vi "testingoutfileopener.vi"() -> ()   [LabVIEW 2020]
doc: "Use this template to build a producer/consumer design pattern. Use this template when you need to execute a process, such as data analysis, when a data source, such as a triggered acquisition, produces data at an uneven rate and you need to execute the process when the data becomes available.\n------------------------------------\nAuther: Koji Ohashi\nCopyright (c) 2020 Japan LabVIEW Users Group, Volunteer members.\nThis VI is released under the MIT License.\nhttp://opensource.org/licenses/mit-license.php\n------------------------------------"
uses:
  For fsr type def.ctl
  <vilib>/Analysis/baseanly.llb/Mean (DBL).vi
  <vilib>/Instr/_visa.llb/VISA Configure Serial Port (Instr).vi
  <vilib>/Analysis/NI_AALBase.lvlib
panel:
  in  "Folder name: Participant":string caption="Participant Name (FirstLast)"
  in  "Create/Replace file":bool
  out "Vout F4":dbl(slide) scale=0.0..5.0
  out "Collecting":bool
  in  "Timer [ms]":u32=5000
  out "On Time [ms]":u32
  out "millisecond timer":u32
  in  "Weight":T1(ring)
  out "Vout F1":dbl(slide) scale=0.0..5.0
  in  "Refresh":bool
  in  "Test Type":string
  in  "Path":path=path "C:/Users/rsKite/Documents/FSR DATA"
  in  "Trial":string caption="Participant Name (FirstLast)"
  out "File Name":string
  out "Vout F3":dbl(slide) scale=0.0..5.0
  out "Vout F2":dbl(slide) scale=0.0..5.0
  out "Status":string
  in  "Collect":bool
  in  "VISA resource name":refnum<visa-resource-name>="COM1"
  in  "stop":bool
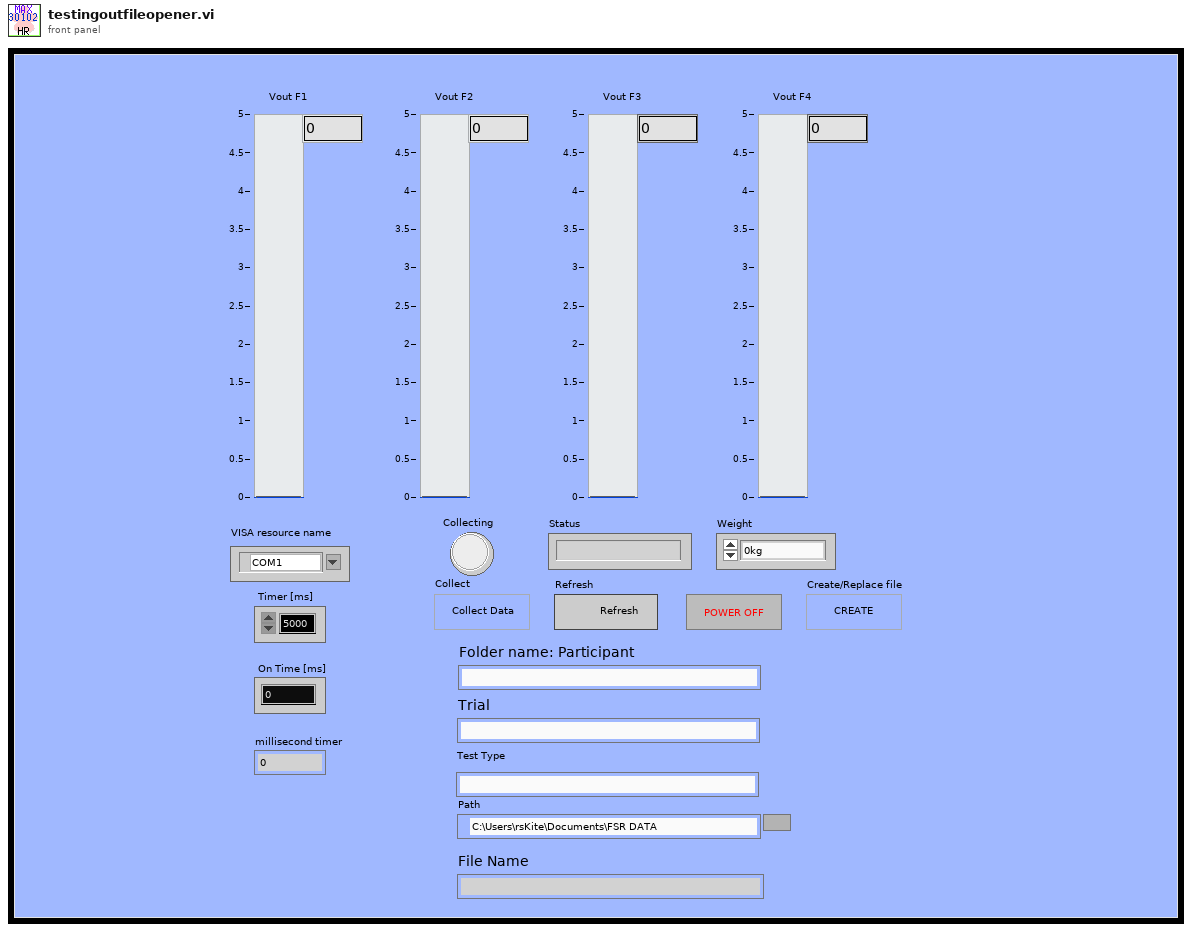
[diagram p1: front panel]
types:
  T1 = enum16{"0kg", "0.1kg", "0.2kg", "0.3kg", "0.4kg", "0.5kg", "0.6kg", "0.7kg", "0.8kg", "0.9kg", "1kg", "1.1kg", "1.2kg", "1.3kg", "1.4kg", "1.5kg", "1.6kg", "1.7kg", "1.8kg", "1.9kg", "2.0kg"}
  T2 = typedef "For fsr type def.ctl" = enum16{"Create/Replace File", "Waiting Room", "Collect Data", "Write Data", "Close File", "Reinit"}
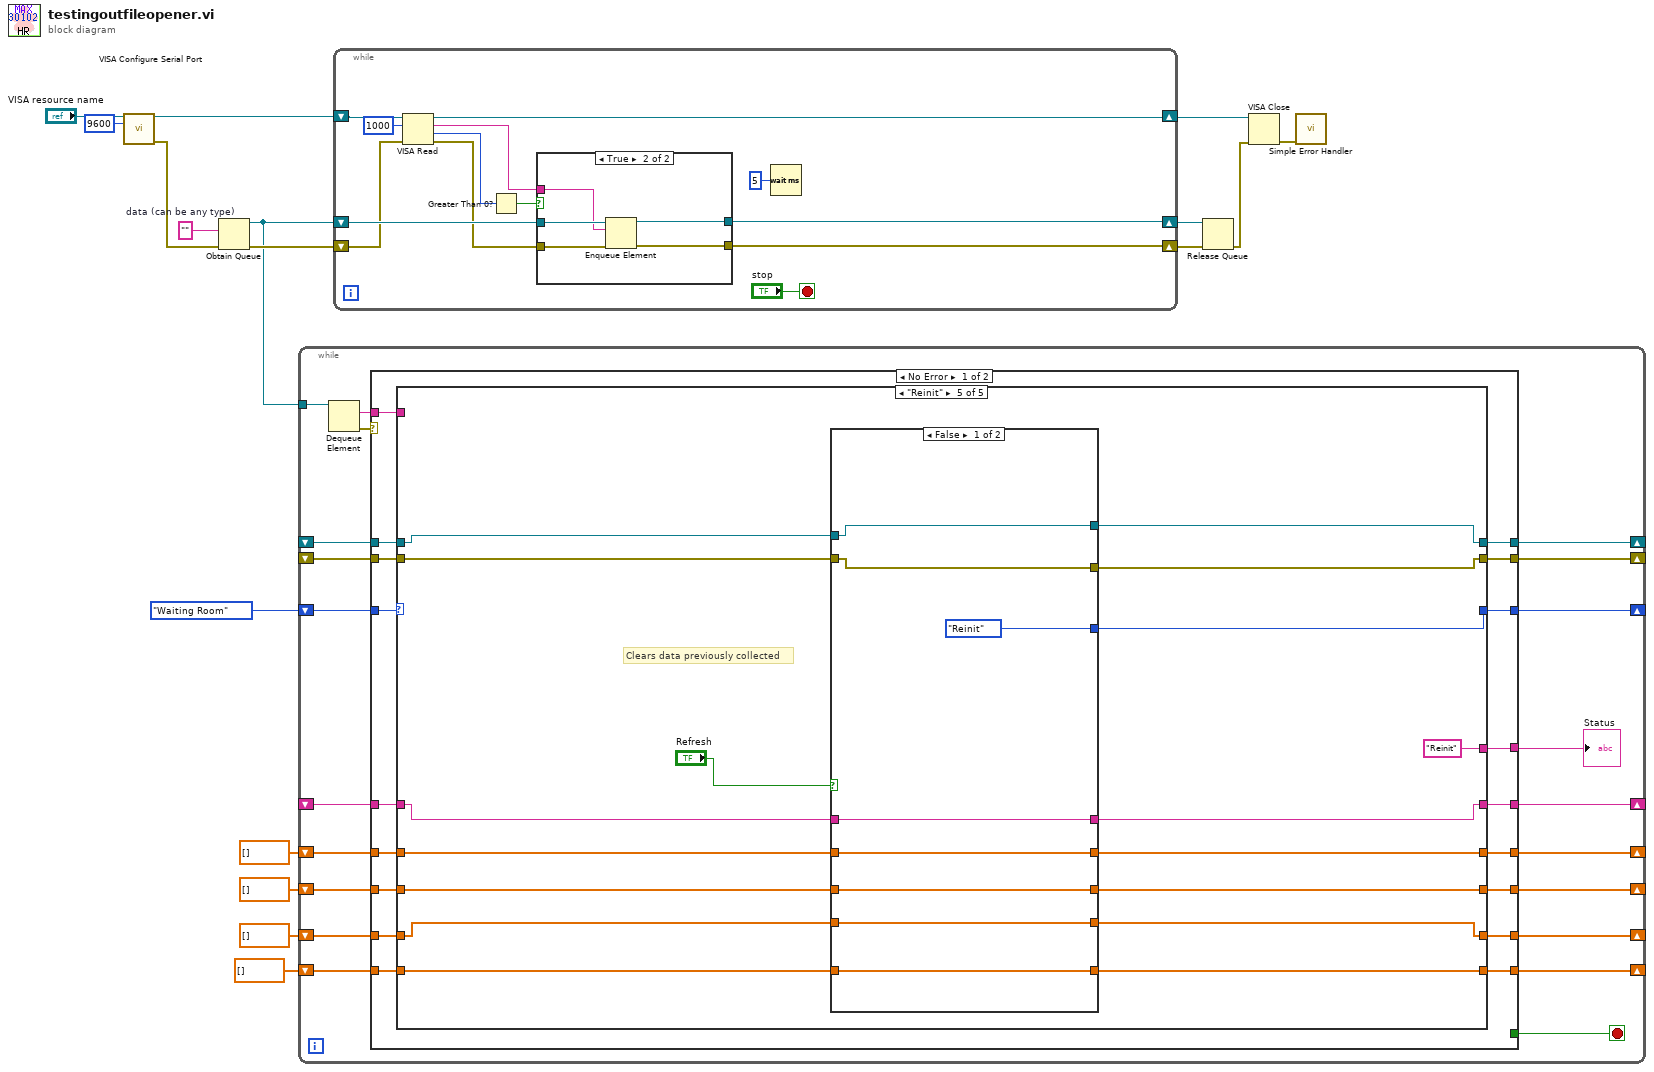
[diagram p0: block diagram]
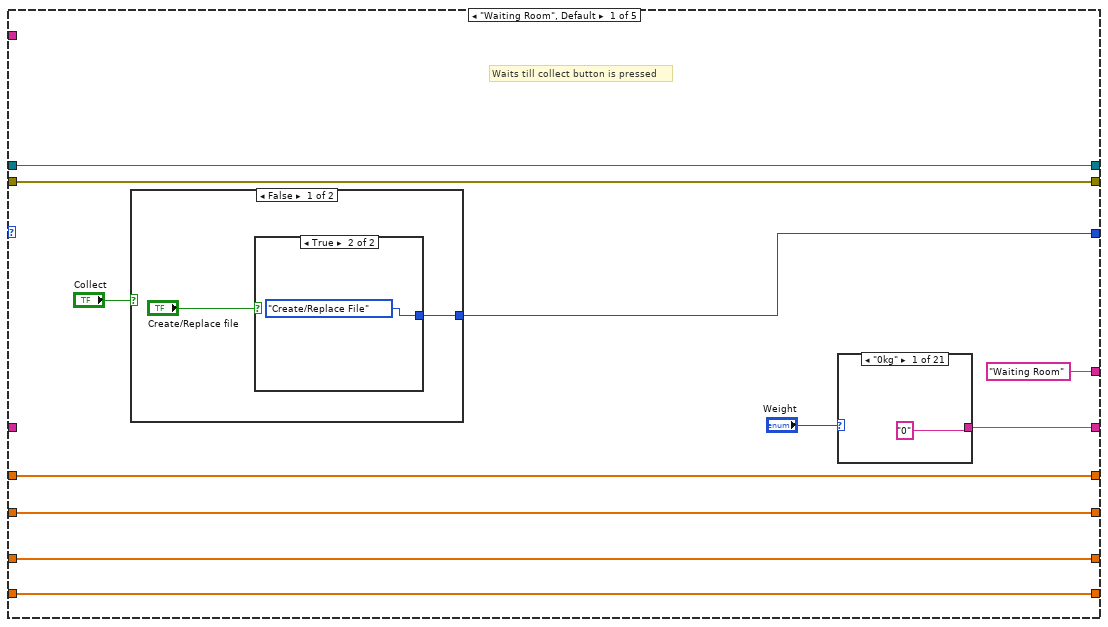
[diagram p2: hidden frame]
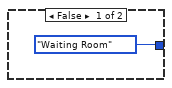
[diagram p3: hidden frame]
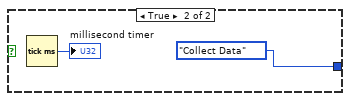
[diagram p4: hidden frame]
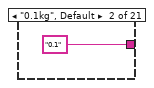
[diagram p5: hidden frame]
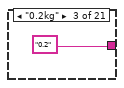
[diagram p6: hidden frame]
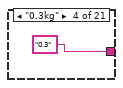
[diagram p7: hidden frame]
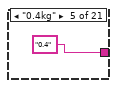
[diagram p8: hidden frame]
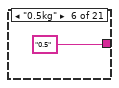
[diagram p9: hidden frame]
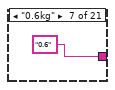
[diagram p10: hidden frame]
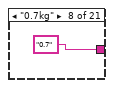
[diagram p11: hidden frame]
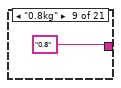
[diagram p12: hidden frame]
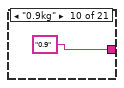
[diagram p13: hidden frame]
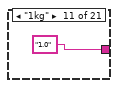
[diagram p14: hidden frame]
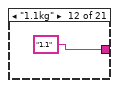
[diagram p15: hidden frame]
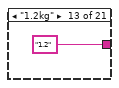
[diagram p16: hidden frame]
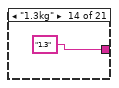
[diagram p17: hidden frame]
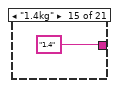
[diagram p18: hidden frame]
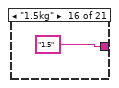
[diagram p19: hidden frame]
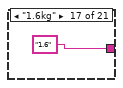
[diagram p20: hidden frame]
diagram:
  w14 = ""  # data (can be any type)
  n1 = call-poly "VISA Configure Serial Port"("VISA resource name"="VISA resource name", "baud rate (9600)"=u32 9600) -> ("VISA resource name out"=w12:refnum<visa-resource-name>, "error out"=w9:errorcluster)  [unwired: 8 in, 4 out]
  n2 = Obtain Queue(element data type=w14, error in (no error)=w9) -> (queue out=w1:refnum<queue>, error out=w17:errorcluster)  [unwired: 3 in, 1 out]
  n3 = while {
    tunnel: w1 -> [w38]
    shift-right: [w33] -> _
    shift-left: For_fsr_type_def."Waiting Room" -> [w34]
    shift-right: [w29] -> _
    shift-left: dbl[] [] -> [w30]
    shift-right: [w31] -> _
    shift-left: dbl[] [] -> [w32]
    shift-right: [w27] -> _
    shift-left: dbl[] [] -> [w28]
    shift-right: [w25] -> _
    shift-left: _ -> [w26]
    shift-right: [w23] -> _
    shift-left: dbl[] [] -> [w24]
    shift-right: [w21] -> _
    shift-left: _ -> [w19]
    shift-right: [w20] -> _
    shift-left: _ -> [w18]
    stop <- w22 stop-if-true
    n4 = Dequeue Element(queue=w38) -> (element=w36:string, error out=w37:errorcluster)  [unwired: 2 in, 2 out]
    n5 = case shown="No Error" w37 {
      tunnel: w36 -> [w54 _]
      tunnel: [w53 "Error or POWER OFF"] -> w35
      tunnel: w34 -> [w56 _]
      tunnel: [w55 For_fsr_type_def."Waiting Room"] -> w33
      tunnel: w32 -> [w52 w213]
      tunnel: [w51 w213] -> w31
      tunnel: w30 -> [w50 w214]
      tunnel: [w49 w214] -> w29
      tunnel: w28 -> [w48 w215]
      tunnel: [w47 w215] -> w27
      tunnel: w26 -> [w46 w212]
      tunnel: [w45 w212] -> w25
      tunnel: w24 -> [w44 w211]
      tunnel: [w43 w211] -> w23
      tunnel: [_ TRUE] -> w22
      tunnel: [w42 w209] -> w21
      tunnel: [w41 w208] -> w20
      tunnel: w19 -> [w40 w209]
      tunnel: w18 -> [w39 w208]
      frame No Error {
        n6 = case shown="\"Reinit\"" w56 {
          tunnel: [w59 For_fsr_type_def."Waiting Room" w112 For_fsr_type_def."Reinit" w184] -> w55
          tunnel: w54 -> [_ _ w138 _ _]
          tunnel: ["Waiting Room" "Creating" "Collect data" "Write Data" "Reinit"] -> w53
          tunnel: w52 -> [w64 w98 w134 w162 w179]
          tunnel: [w64 w98 w119 w162 w188] -> w51
          tunnel: w50 -> [w65 w99 w131 w163 w180]
          tunnel: [w65 w99 w129 w163 w187] -> w49
          tunnel: w48 -> [w66 w101 w130 w164 w181]
          tunnel: [w66 w101 w128 w164 w186] -> w47
          tunnel: [w63 w100 w126 w154 w185] -> w45
          tunnel: w46 -> [_ w100 w126 w154 w182]
          tunnel: w44 -> [w61 w97 w117 w153 w178]
          tunnel: [w61 w97 w116 w153 w189] -> w43
          tunnel: [w58 w105 w110 w145 w174] -> w42
          tunnel: [w57 w104 w109 w144 w175] -> w41
          tunnel: w40 -> [w58 _ w110 w147 w177]
          tunnel: w39 -> [w57 _ w109 w146 w176]
          frame "Waiting Room", Default {
            # "Waits till collect button is pressed"
            n7 = case shown="False" "Collect" {
              tunnel: [w68 For_fsr_type_def."Collect Data"] -> w59
              frame False {
                n8 = case shown="True" "Create/Replace file" {
                  tunnel: [For_fsr_type_def."Waiting Room" For_fsr_type_def."Create/Replace File"] -> w68
                  frame False {
                  }
                  frame True {
                  }
                }
              }
              frame True {
                n9 = Tick Count (ms)() -> (millisecond timer value=→"millisecond timer":u32)
              }
            }
            n10 = case shown="\"0kg\"" "Weight" {
              tunnel: ["0" "0.1" "0.2" "0.3" "0.4" "0.5" "0.6" "0.7" "0.8" "0.9" "1.0" "1.1" "1.2" "1.3" "1.4" "1.5" "1.6" "1.7" "1.8" "1.9" "2.0"] -> w63
              frame "0kg" {
              }
              frame "0.1kg", Default {
              }
              frame "0.2kg" {
              }
              frame "0.3kg" {
              }
              frame "0.4kg" {
              }
              frame "0.5kg" {
              }
              frame "0.6kg" {
              }
              frame "0.7kg" {
              }
              frame "0.8kg" {
              }
              frame "0.9kg" {
              }
              frame "1kg" {
              }
              frame "1.1kg" {
              }
              frame "1.2kg" {
              }
              frame "1.3kg" {
              }
              frame "1.4kg" {
              }
              frame "1.5kg" {
              }
              frame "1.6kg" {
              }
              frame "1.7kg" {
              }
              frame "1.8kg" {
              }
              frame "1.9kg" {
              }
              frame "2.0kg" {
              }
            }
          }
          frame "Create/Replace File" {
            n11 = call "fileSUB.vi"("Folder name: Participant"="Folder name: Participant", "Weight"="Test Type", "Trial"="Trial", "Path"="Path") -> ("error out"=w104:errorcluster, "refnum out"=w105:refnum<file>, "File Name"=→"File Name":string)  [unwired: 5 in]
          }
          frame "Collect Data" {
            w120 = ","
            # "Collects data from Arduino\n Stops when timer is up"
            n12 = Match Pattern(string=w138, regular expression=w120) -> (before substring=w136:string, after substring=w135:string)  [unwired: 1 in, 2 out]
            n13 = Match Pattern(string=w135, regular expression=w120) -> (before substring=w137:string, after substring=w115:string)  [unwired: 1 in, 2 out]
            n14 = Fract/Exp String To Number(string=w136) -> (number=w127:dbl)  [unwired: 3 in, 1 out]
            "Vout F1" <- w127
            n15 = Match Pattern(string=w115, regular expression=w120) -> (before substring=w114:string, after substring=w121:string)  [unwired: 1 in, 2 out]
            n16 = Fract/Exp String To Number(string=w137) -> (number=w132:dbl)  [unwired: 3 in, 1 out]
            "Vout F2" <- w132
            n17 = Fract/Exp String To Number(string=w121) -> (number=w118:dbl)  [unwired: 3 in, 1 out]
            "Vout F4" <- w118
            n18 = Fract/Exp String To Number(string=w114) -> (number=w133:dbl)  [unwired: 3 in, 1 out]
            "Vout F3" <- w133
            n19 = Build Array (concatenate)(w130, w127) -> (w128:dbl[])
            n20 = Build Array (concatenate)(w134, w133) -> (w119:dbl[])
            n21 = Build Array (concatenate)(w131, w132) -> (w129:dbl[])
            n22 = Build Array (concatenate)(w117, w118) -> (w116:dbl[])
            n23 = local read "millisecond timer"() -> (w122:u32)
            n24 = Tick Count (ms)() -> (millisecond timer value=w125:u32)
            n25 = Subtract(x=w125, y=w122) -> (x-y=w124:u32)
            "On Time [ms]" <- w124
            n26 = Greater?(x=w124, y="Timer [ms]") -> (0:w111:bool)
            n27 = case shown="True" w111 {
              tunnel: [TRUE ("Collecting") FALSE ("Collecting")] -> w113
              tunnel: [For_fsr_type_def."Collect Data" For_fsr_type_def."Write Data"] -> w112
              frame False {
              }
              frame True {
              }
            }
            "Collecting" <- w113
          }
          frame "Write Data" {
            # "Puts the data to a spreadsheet and writes it to the file"
            n28 = call-poly <vilib>:"Mean.vi"("X"=w164) -> ("mean"=w161:dbl)  [unwired: 1 out]
            n29 = call-poly <vilib>:"Mean.vi"("X"=w163) -> ("mean"=w160:dbl)  [unwired: 1 out]
            n30 = call-poly <vilib>:"Mean.vi"("X"=w162) -> ("mean"=w159:dbl)  [unwired: 1 out]
            n31 = call-poly <vilib>:"Mean.vi"("X"=w153) -> ("mean"=w152:dbl)  [unwired: 1 out]
            n32 = Build Array(w161, w160, w159, w152) -> (w157:dbl[])
            n33 = Reshape Array(w157, 4 ("dimension size")) -> (w158:dbl[])
            n34 = Array To Spreadsheet String(array=w158, 3:"%5.3f" ("format string")) -> (spreadsheet string=w148:string)  [unwired: 1 in]
            n35 = Concatenate Strings(w154, "\r\n", "F1", "\t", "F2", "\t", "F3", "\t", "F4", "\r\n", w148) -> (w170:string)
            n36 = Write to Text File(file (use dialog)=w147, text=w170, error in=w146) -> (refnum out=w145:refnum<file>, error out=w144:errorcluster)  [unwired: 1 in, 1 out]
          }
          frame "Reinit" {
            # "Clears data previously collected"
            n37 = case shown="False" "Refresh" {
              tunnel: [w194 dbl[] []] -> w189
              tunnel: [w195 dbl[] []] -> w188
              tunnel: [w196 dbl[] []] -> w187
              tunnel: [w197 dbl[] []] -> w186
              tunnel: [w198 ""] -> w185
              tunnel: [For_fsr_type_def."Reinit" For_fsr_type_def."Waiting Room"] -> w184
              tunnel: w182 -> [w198 _]
              tunnel: w181 -> [w197 _]
              tunnel: w180 -> [w196 _]
              tunnel: w179 -> [w195 _]
              tunnel: w178 -> [w194 _]
              tunnel: w177 -> [w192 w199]
              tunnel: w176 -> [w191 w201]
              tunnel: [w191 w200] -> w175
              tunnel: [w192 w199] -> w174
              frame False {
              }
              frame True {
                n38 = Close File(refnum=w199, error in=w201) -> (error out=w200:errorcluster)  [unwired: 1 out]
                n39 = call <vilib>:"General Error Handler.vi"("error in (no error)"=w200) -> ()  [unwired: 10 in, 5 out]
              }
            }
          }
        }
      }
      frame Error {
      }
    }
    "Status" <- w35
  }
  n40 = while {
    shift-right: [w227] -> w15
    shift-left: w17 -> [w221]
    shift-right: [w228] -> w16
    shift-left: w1 -> [w229]
    shift-right: [w225] -> w10
    shift-left: w12 -> [w219]
    stop <- "stop" stop-if-true
    n41 = VISA Read(VISA resource name=w219, byte count=u32 1000, error in (no error)=w221) -> (VISA resource name out=w225:refnum<visa-resource-name>, read buffer=w222:string, return count=w224:u32, error out=w220:errorcluster)
    n42 = Greater Than 0?(x=w224) -> (x > 0?=w223:bool)
    n43 = case shown="True" w223 {
      tunnel: w229 -> [w232 w237]
      tunnel: [w232 w236] -> w228
      tunnel: w220 -> [w231 w235]
      tunnel: [w231 w234] -> w227
      tunnel: w222 -> [_ w233]
      frame False {
      }
      frame True {
        n44 = Enqueue Element(queue=w237, element=w233, error in (no error)=w235) -> (queue out=w236:refnum<queue>, error out=w234:errorcluster)  [unwired: 1 in, 1 out]
      }
    }
    n45 = Wait (ms)(milliseconds to wait=u32 5) -> ()  [unwired: 1 out]
  }
  n46 = Release Queue(queue=w16, error in (no error)=w15) -> (error out=w8:errorcluster)  [unwired: 1 in, 2 out]
  n47 = VISA Close(VISA resource name=w10, error in (no error)=w8) -> (error out=w11:errorcluster)
  n48 = call <vilib>:"Simple Error Handler.vi"("error in (no error)"=w11) -> ()  [unwired: 1 in, 8 out]
